vi "Zadanie 4.vi"() -> ()   [LabVIEW 2020]
panel:
  out "XY Graph 2":cluster{i32[], dbl[]}[](graph)
  in  "Zmiana Wartoœci krytycznej 2":dbl(slide) scale=0.0..10.0
  in  "Zmiana Wartoœci krytycznej":dbl(slide) scale=0.0..10.0
  out "XY Graph":cluster{dbl[], dbl[]}[](graph)
  in  "stop":bool
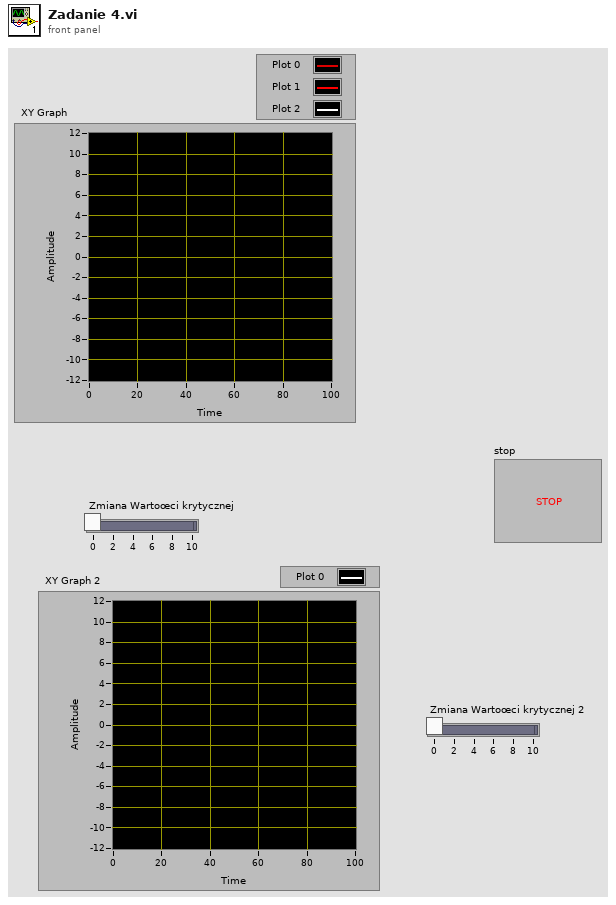
[diagram p1: front panel]
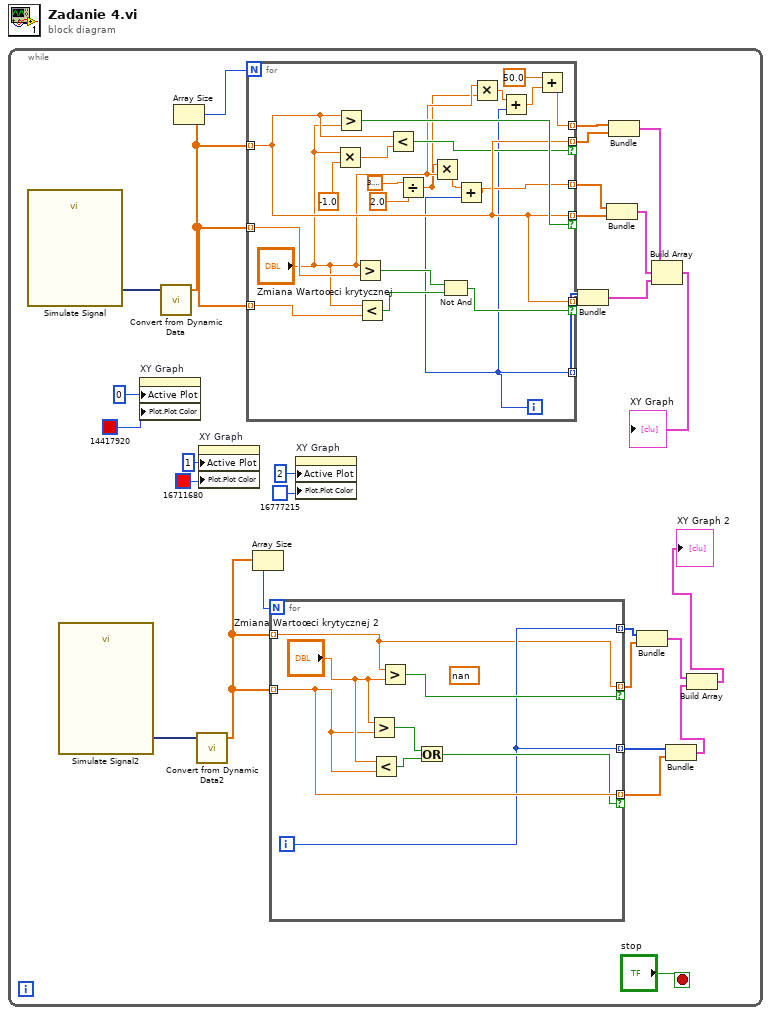
[diagram p0: block diagram]
diagram:
  n1 = while {
    stop <- "stop" stop-if-true
    n2 = call "Simulate Signal"() -> ("Sine with Uniform Noise"=w29:dynamicdata)  [unwired: 14 in, 1 out]
    n3 = call "Simulate Signal2"() -> ("Sine with Uniform Noise"=w10:dynamicdata)  [unwired: 14 in, 1 out]
    n4 = property on="XY Graph" class="XYGraph (strict)"("Active Plot"=u32 0, "Plot.Plot Color"=u32 14417920) -> ()  [unwired: 2 in, 2 out]
    n5 = call "Convert from Dynamic Data"("Dynamic Data Type"=w29) -> ("Array"=w23:dbl[])  [unwired: 3 in]
    n6 = Array Size(array=w23) -> (size(s)=w28:i32)
    n7 = call "Convert from Dynamic Data2"("Dynamic Data Type"=w10) -> ("Array"=w7:dbl[])  [unwired: 3 in]
    n8 = property on="XY Graph" class="XYGraph (strict)"("Active Plot"=u32 1, "Plot.Plot Color"=u32 16711680) -> ()  [unwired: 2 in, 2 out]
    n9 = for {
      N: w28 -> [_]
      tunnel: w23 -> [w53] mode=indexing
      tunnel: [w53] -> w24 mode=indexing if=w54
      tunnel: [w43] -> w21 mode=indexing
      tunnel: w23 -> [w56] mode=indexing
      tunnel: w23 -> [w55] mode=indexing
      tunnel: [w53] -> w22 mode=indexing if=w57
      tunnel: [w49] -> w19 mode=indexing
      tunnel: [w40] -> w15 mode=indexing
      tunnel: [w53] -> w14 mode=indexing if=w52
      i -> [w43]
      n10 = Multiply(x="Zmiana Wartoœci krytycznej", y=-1.0) -> (x*y=w50:dbl)
      n11 = Greater?(x=w53, y="Zmiana Wartoœci krytycznej") -> (0:w54:bool)
      n12 = Greater?(x="Zmiana Wartoœci krytycznej", y=w56) -> (0:w59:bool)
      n13 = Less?(x="Zmiana Wartoœci krytycznej", y=w55) -> (x < y?=w58:bool)
      n14 = Less?(x=w53, y=w50) -> (x < y?=w52:bool)
      n15 = Divide(x=3.141592653589793, y=2.0) -> (x/y=w39:dbl)
      n16 = Multiply(x=w39, y="Zmiana Wartoœci krytycznej") -> (x*y=w48:dbl)
      n17 = Not And(1:w58, 2:w59) -> (0:w57:bool)
      n18 = Add(x=w48, y=w43) -> (x+y=w49:dbl)
      n19 = Multiply(x="Zmiana Wartoœci krytycznej", y=w39) -> (x*y=w44:dbl)
      n20 = Add(x=w44, y=w43) -> (x+y=w41:dbl)
      n21 = Add(x=50.0, y=w41) -> (x+y=w40:dbl)
    }
    n22 = Array Size(array=w7) -> (size(s)=w9:i32)
    n23 = for {
      N: w9 -> [_]
      tunnel: w7 -> [w31] mode=indexing
      tunnel: [w31] -> w2 mode=indexing if=w38
      tunnel: [w32] -> w8 mode=indexing
      tunnel: w7 -> [w34] mode=indexing
      tunnel: [w34] -> w6 mode=indexing if=w33
      tunnel: [w32] -> w5 mode=indexing
      i -> [w32]
      (unwired) nan
      n24 = Greater?(x="Zmiana Wartoœci krytycznej 2", y=w34) -> (0:w36:bool)
      n25 = Less?(x="Zmiana Wartoœci krytycznej 2", y=w34) -> (x < y?=w35:bool)
      n26 = Greater?(x=w31, y="Zmiana Wartoœci krytycznej 2") -> (0:w38:bool)
      n27 = Or(x=w36, y=w35) -> (x .or. y?=w33:bool)
    }
    n28 = property on="XY Graph" class="XYGraph (strict)"("Active Plot"=u32 2, "Plot.Plot Color"=u32 16777215) -> ()  [unwired: 2 in, 2 out]
    n29 = Bundle(w21, w22) -> (w25:cluster{i32[], dbl[]})  [unwired: 1 in]
    n30 = Bundle(w19, w24) -> (w26:cluster{dbl[], dbl[]})  [unwired: 1 in]
    n31 = Bundle(w15, w14) -> (w13:cluster{dbl[], dbl[]})  [unwired: 1 in]
    n32 = Bundle(w8, w2) -> (w1:cluster{i32[], dbl[]})  [unwired: 1 in]
    n33 = Build Array(w13, w26, w25) -> (→"XY Graph":cluster{dbl[], dbl[]}[])
    n34 = Bundle(w5, w6) -> (w4:cluster{i32[], dbl[]})  [unwired: 1 in]
    n35 = Build Array(w1, w4) -> (→"XY Graph 2":cluster{i32[], dbl[]}[])
  }
